vi "AMZ_S3_APIHLP_Convert Byte Range to Range Header.vi"(4 "Range":T2) -> (1 "HTTP Header-Value pair":T1={"Header"="User-Agent", "Value"=""})   [LabVIEW 2015, in "LV Interface for Amazon S3.lvlib"]
uses:
  LV Interface for Amazon S3.lvlib
  Typedefs/AMZ_S3_API_GET Request Range.ctl
  Typedefs/AMZ_S3_HTTP Header-Value pair.ctl
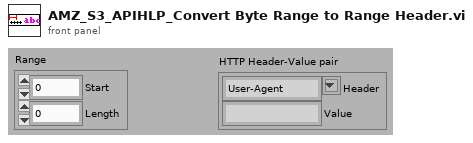
[diagram p1: front panel]
types:
  T1 = typedef "LV Interface for Amazon S3.lvlib/AMZ_S3_HTTP Header-Value pair.ctl" = cluster{"Header":string, "Value":string}
  T2 = typedef "LV Interface for Amazon S3.lvlib/AMZ_S3_API_GET Request Range.ctl" = cluster{"Start":i64, "Length":i64}
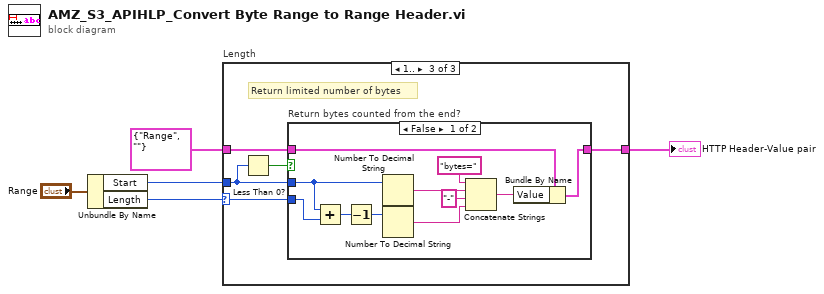
[diagram p0: block diagram]
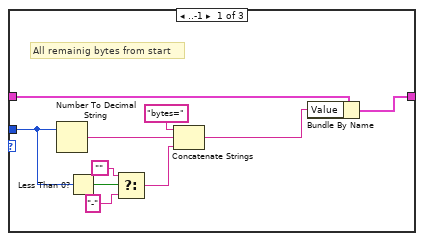
[diagram p2: hidden frame]
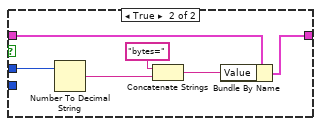
[diagram p4: hidden frame]
diagram:
  n1 = Unbundle By Name("Range") -> ("Start"=w3:i64, "Length"=w4:i64)
  n2 = case "Length" shown="1.." w4 {
    selector: w4 -> [_ _ w20]
    tunnel: w3 -> [w10 _ w19]
    tunnel: T1 {"Header"="Range", "Value"=""} ("HTTP Header-Value pair") -> [w15 w16 w18]
    tunnel: [w14 w16 w17] -> w1
    frame ..-1 {
      # "All remainig bytes from start"
      n3 = Number To Decimal String(number=w10) -> (decimal integer string=w13:string)  [unwired: 1 in]
      n4 = Less Than 0?(x=w10) -> (x < 0?=w9:bool)
      n5 = Select(t="", s=w9, f="-" ("string")) -> (s? t:f=w6:string)
      n6 = Concatenate Strings("bytes=" ("string"), w13, w6) -> (w11:string)
      n7 = Bundle By Name(cluster=w15, "Value"=w11) -> (w14:T1)
    }
    frame 0 {
      # "Return nothing???!!! -> return everything!"
    }
    frame 1.. {
      # "Return limited number of bytes"
      n8 = Less Than 0?(x=w19) -> (x < 0?=w21:bool)
      n9 = case "Return bytes counted from the end?" shown="False" w21 {
        tunnel: w20 -> [w32 _]
        tunnel: w19 -> [w31 w38]
        tunnel: w18 -> [w26 w37]
        tunnel: [w24 w33] -> w17
        frame False {
          n10 = Add(x=w31, y=w32) -> (x+y=w23:i64)
          n11 = Decrement(x=w23) -> (x-1=w22:i64)
          n12 = Number To Decimal String(number=w31) -> (decimal integer string=w30:string)  [unwired: 1 in]
          n13 = Number To Decimal String(number=w22) -> (decimal integer string=w27:string)  [unwired: 1 in]
          n14 = Concatenate Strings("bytes=" ("string"), w30, "-" ("string"), w27) -> (w25:string)
          n15 = Bundle By Name(cluster=w26, "Value"=w25) -> (w24:T1)
        }
        frame True {
          n16 = Number To Decimal String(number=w38) -> (decimal integer string=w36:string)  [unwired: 1 in]
          n17 = Concatenate Strings("bytes=" ("string"), w36) -> (w34:string)
          n18 = Bundle By Name(cluster=w37, "Value"=w34) -> (w33:T1)
        }
      }
    }
  }
  "HTTP Header-Value pair" <- w1
